vi "Load Sub Panel.vi"(8 "error in (no error)":errorcluster, 10 "sub panel":refnum<vi>, 11 "Normal Log in":refnum<class "Normal Log.lvclass">) -> (0 "error out":errorcluster, 3 "Normal Log out":refnum<class "Normal Log.lvclass">)   [LabVIEW 2020, in "Normal Log.lvlib" / "Normal Log.lvclass"]
uses:
  Normal Log.lvclass
  Log/Log Messages/Insert VI Msg/Insert VI Msg.lvclass
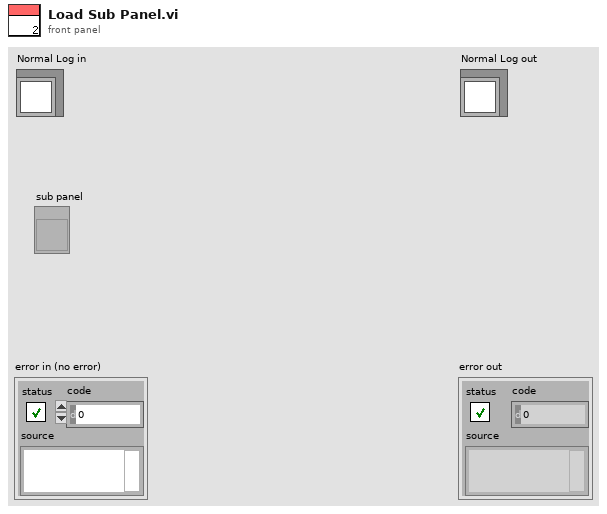
[diagram p1: front panel]
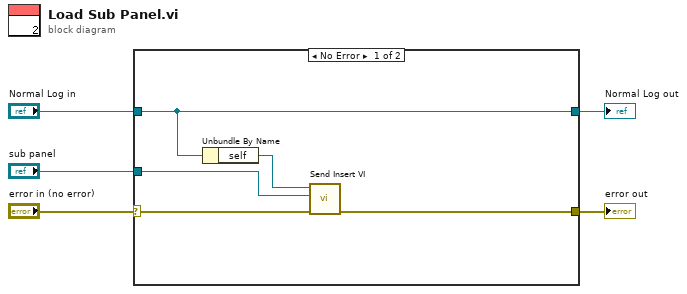
[diagram p0: block diagram]
diagram:
  n1 = case shown="No Error" "error in (no error)" {
    selector: "error in (no error)" -> [w9 w12]
    tunnel: "Normal Log in" -> [w10 w11]
    tunnel: [w6 w12] -> w3
    tunnel: [w10 w11] -> w2
    tunnel: "sub panel" -> [w7 _]
    frame No Error {
      n2 = Unbundle By Name(w10) -> ("self"=w8:refnum<class "Message Enqueuer.lvclass">)
      n3 = call "Send Insert VI.vi"("error in (no error)"=w9, "sub panel"=w7, "Message Enqueuer"=w8) -> ("error out"=w6:errorcluster)  [unwired: 7 in, 1 out]
    }
    frame Error {
    }
  }
  "error out" <- w3
  "Normal Log out" <- w2
